vi "Initialize Globals - Production.vi"(0 "TSM context":T2, 5 "TCs-Common":T1={"SetVDDLevel"=2.5, "Relay Settling Time(s)"=0.0, "J"=0}) -> (15 "error out":errorcluster)   [LabVIEW 2019]
uses:
  <vilib>/NI_TestStand_SemiconductorModule/NI_TestStand_Semiconductor_Module.lvlibp/PinMap/General/SemiconductorModuleContext.ctl
  Common/Utility/typedefs/TCs-Common.ctl
  TSM Context Data Access/TSM Context Data Access.lvclass/TSM Context Data Access.ctl
  Common/Utility/typedefs/TCs-Engineering.ctl
  TSM Context Data Access/Public/Properties/TCs-Common - Write.vi
  TSM Context Data Access/Public/Properties/TCs-Engineering - Write.vi
  <vilib>/NI_TestStand_SemiconductorModule/NI_TestStand_Semiconductor_Module.lvlibp/PinMap/Site and Global Data/SetGlobalData.vi
  TSM Context Data Access/TSM Context Data Access.lvclass
  <vilib>/NI_TestStand_SemiconductorModule/NI_TestStand_Semiconductor_Module.lvlibp
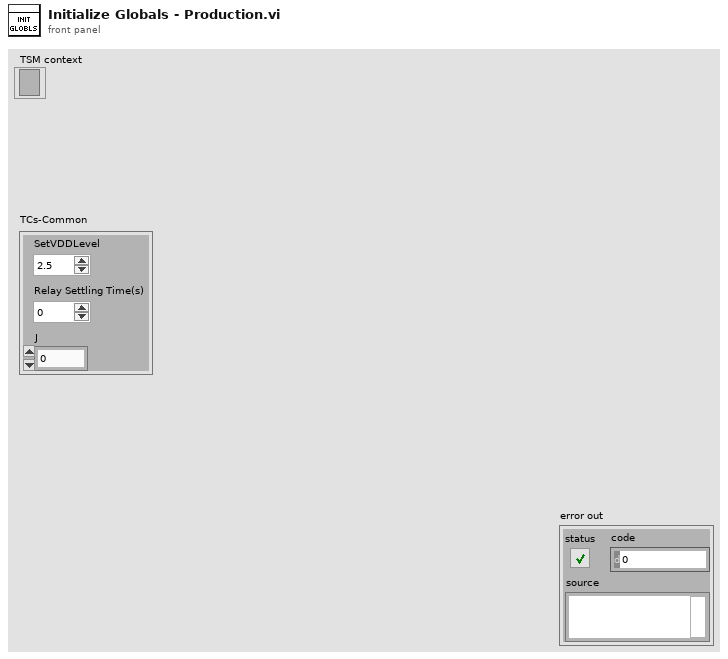
[diagram p1: front panel]
types:
  T1 = typedef "TCs-Common.ctl" = cluster{"SetVDDLevel":dbl, "Relay Settling Time(s)":dbl, "J":i8}
  T2 = typedef "NI_TestStand_Semiconductor_Module.lvlibp/SemiconductorModuleContext.ctl" = refnum<k7>
  T3 = typedef "TCs-Engineering.ctl" = cluster{"Disable Fuses Blow":bool, "Disable Master Fuse Blow":bool}
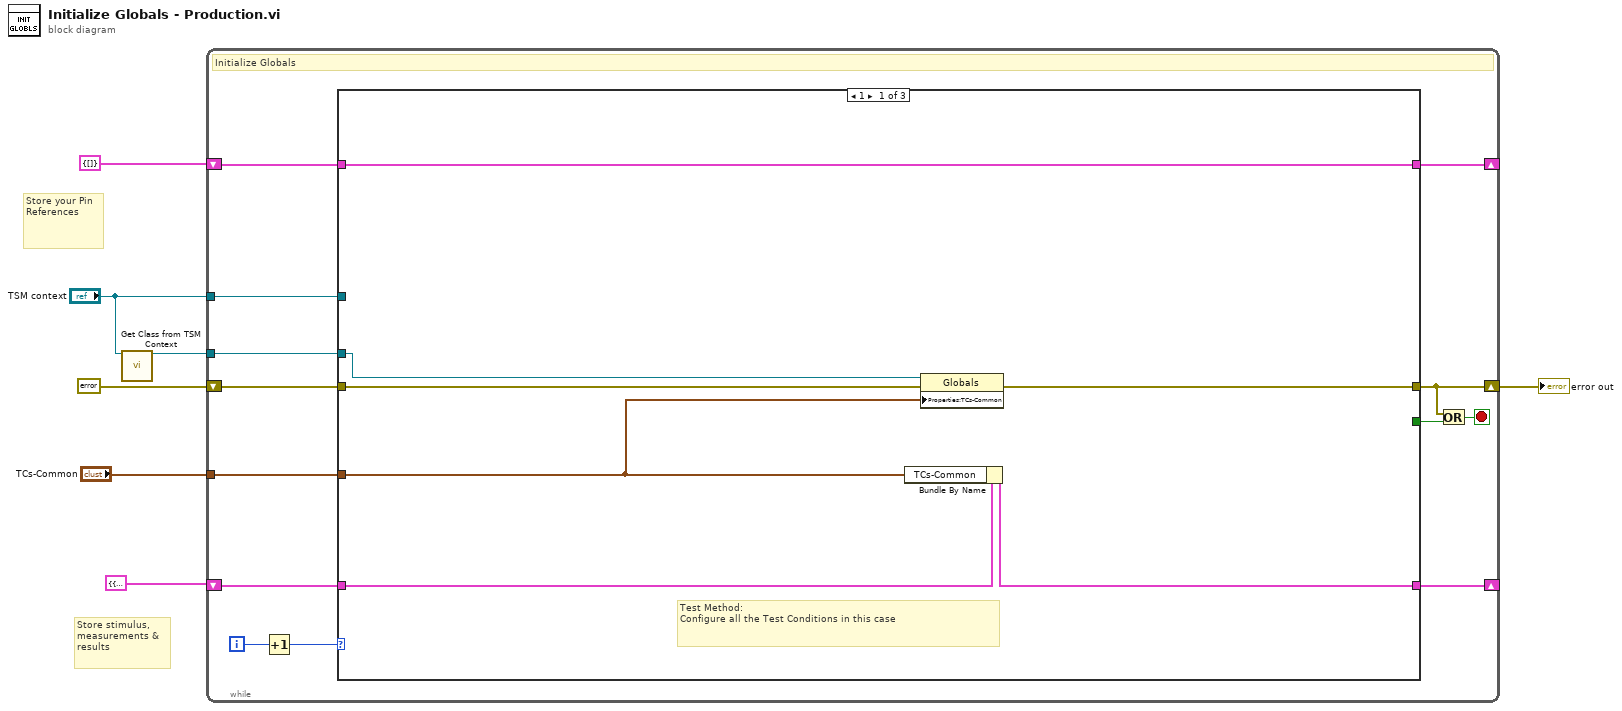
[diagram p0: block diagram]
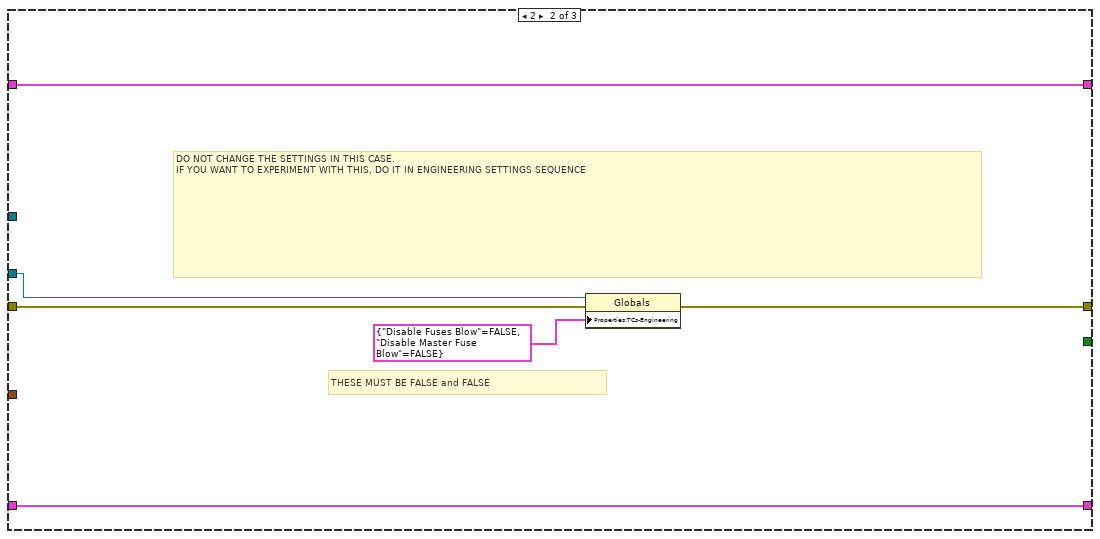
[diagram p2: hidden frame]
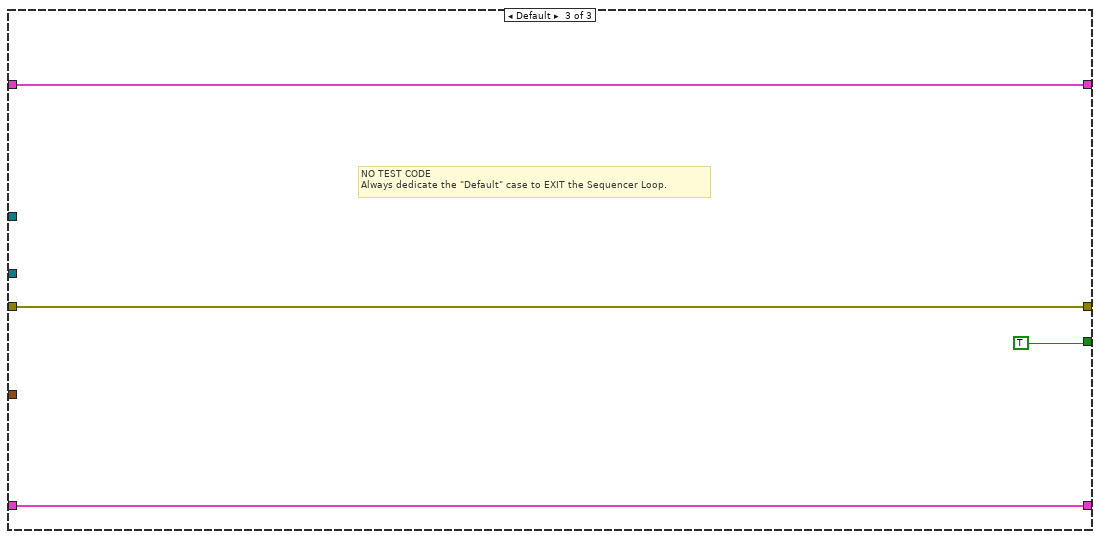
[diagram p3: hidden frame]
diagram:
  # "Store stimulus, measurements & results"
  # "Store your Pin References"
  n1 = call "Get Class from TSM Context.vi"("TSM Context"="TSM context") -> ("Global Memory Class"=w2:refnum<class "TSM Context Data Access.lvclass">)  [unwired: 14 in]
  n2 = while {
    shift-right: [w12] -> w7
    shift-left: errorcluster {"status"=FALSE, "code"=0, "source"=""} ("error in") -> [w19]
    tunnel: "TSM context" -> [w17]
    shift-right: [w14] -> _
    shift-left: cluster{"Site Numbers":i32[]} {"Site Numbers"=[]} -> [w15]
    shift-right: [w11] -> _
    shift-left: cluster{"TCs-Common":T1} {"TCs-Common"={"SetVDDLevel"=2.5, "Relay Settling Time(s)"=0.0, "J"=0}} ("TCs") -> [w10]
    tunnel: w2 -> [w9]
    tunnel: "TCs-Common" -> [w8]
    i -> [w20]
    stop <- w13 stop-if-true
    # "Initialize Globals"
    n3 = Increment(x=w20) -> (x+1=w18:i32)
    n4 = case shown="1" w18 {
      tunnel: [w22 w30 w36] -> w12
      tunnel: w19 -> [w23 w31 w36]
      tunnel: w17 -> [_ _ _]
      tunnel: [_ _ TRUE] -> w16
      tunnel: w15 -> [w27 w33 w35]
      tunnel: [w27 w33 w35] -> w14
      tunnel: [w25 w29 w34] -> w11
      tunnel: w10 -> [w26 w29 w34]
      tunnel: w9 -> [w24 w32 _]
      tunnel: w8 -> [w21 _ _]
      frame 1 {
        # "Test Method:\nConfigure all the Test Conditions in this case"
        # "Test Conditions and Instrument Settings"
        n5 = Bundle By Name(cluster=w26, "TCs-Common"=w21) -> (w25:cluster{"TCs-Common":T1})
        n6 = property class="Globals"(reference=w24, error in=w23, "Properties:TCs-Common"=w21) -> (error out=w22:errorcluster)  [unwired: 1 out]
      }
      frame 2 {
        # "THESE MUST BE FALSE and FALSE"
        # "DO NOT CHANGE THE SETTINGS IN THIS CASE.\nIF YOU WANT TO EXPERIMENT WITH THIS, DO IT IN ENGINEERING SETTINGS SEQUENCE"
        # "Test Conditions and Instrument Settings"
        n7 = property class="Globals"(reference=w32, error in=w31, "Properties:TCs-Engineering"=T3 {"Disable Fuses Blow"=FALSE, "Disable Master Fuse Blow"=FALSE} ("TCs-Engineering")) -> (error out=w30:errorcluster)  [unwired: 1 out]
      }
      frame Default {
        # "NO TEST CODE\nAlways dedicate the \"Default\" case to EXIT the Sequencer Loop."
        # "Exit Loop"
      }
    }
    n8 = Or(x=w12, y=w16) -> (x .or. y?=w13:bool)
  }
  "error out" <- w7
